vi "Puzzle 7-1.vi"() -> ()   [LabVIEW 2022 SP3]
uses:
  <vilib>/Analysis/NI_AALBase.lvlib
panel:
  in  "delimited string":string="Time:        53     71     78     80\nDistance:   275   1181   1215   1524"
  out "Numeric":i64
  out "Array":T1(array[ring])
  out "logical OR":bool
  out "Hands sorted":T2(array[cluster])
  out "Hands identified":T2(array[cluster])
  out "Map":map{string, u8}(c390)
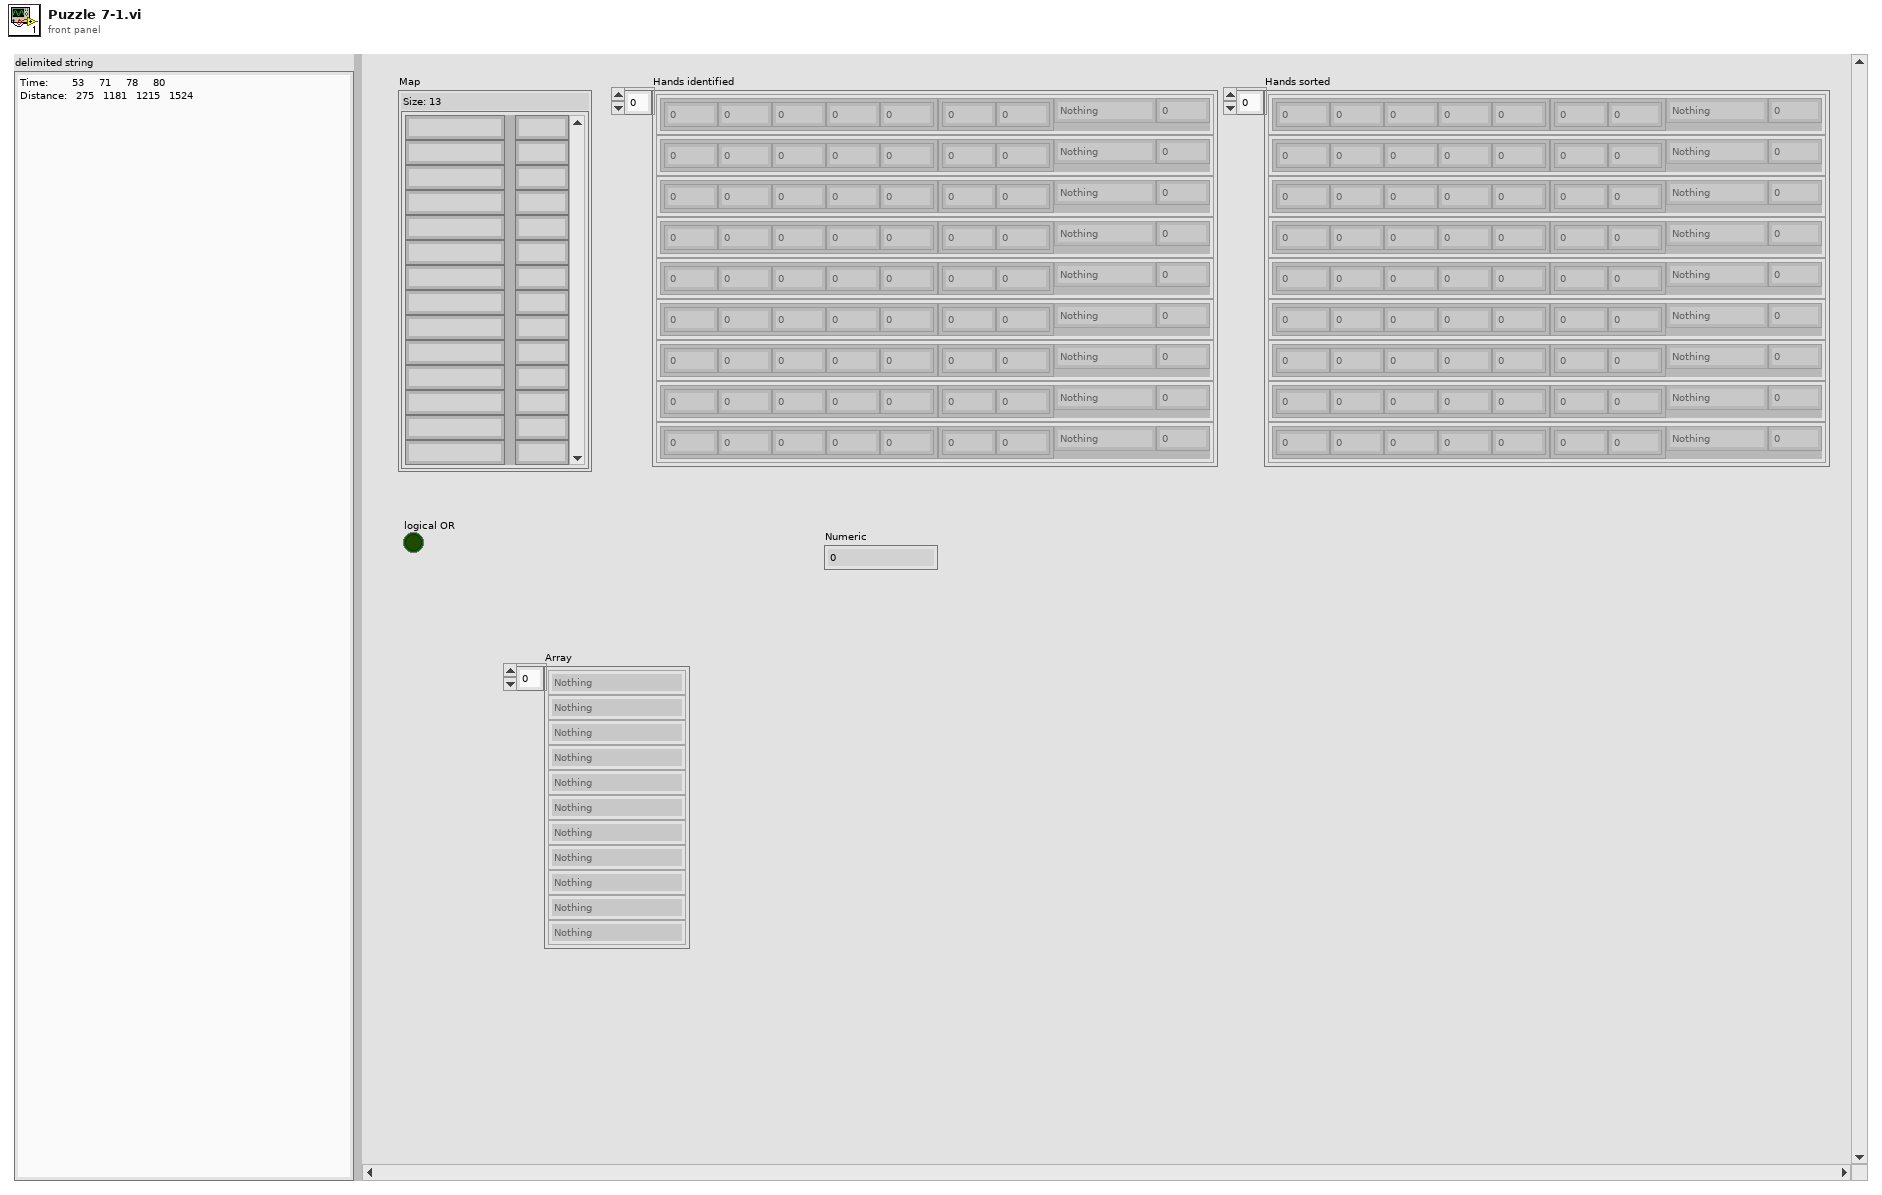
[diagram p1: front panel]
types:
  T1 = enum16{"Nothing", "One Pair", "Two Pair", "Three of a Kind", "Full House", "Four of a Kind", "Five of a Kind"}[]
  T2 = cluster{u8[], cluster{"size":i32, i32}, "value":enum16{"Nothing", "One Pair", "Two Pair", "Three of a Kind", "Full House", "Four of a Kind", "Five of a Kind"}, i32}[]
  T3 = map{enum16{"Nothing", "One Pair", "Two Pair", "Three of a Kind", "Full House", "Four of a Kind", "Five of a Kind"}, set{cluster{u8[], cluster{"size":i32, i32}, "value":enum16{"Nothing", "One Pair", "Two Pair", "Three of a Kind", "Full House", "Four of a Kind", "Five of a Kind"}, i32}}}
  T4 = enum16{"Nothing", "One Pair", "Two Pair", "Three of a Kind", "Full House", "Four of a Kind", "Five of a Kind"}
  T5 = map{cluster{"size of set":i32, "histogram max":i32}, enum16{"Nothing", "One Pair", "Two Pair", "Three of a Kind", "Full House", "Four of a Kind", "Five of a Kind"}}
  T6 = cluster{u8[], cluster{"size":i32, i32}, "value":enum16{"Nothing", "One Pair", "Two Pair", "Three of a Kind", "Full House", "Four of a Kind", "Five of a Kind"}, i32}
  T7 = set{cluster{u8[], cluster{"size":i32, i32}, "value":enum16{"Nothing", "One Pair", "Two Pair", "Three of a Kind", "Full House", "Four of a Kind", "Five of a Kind"}, i32}}
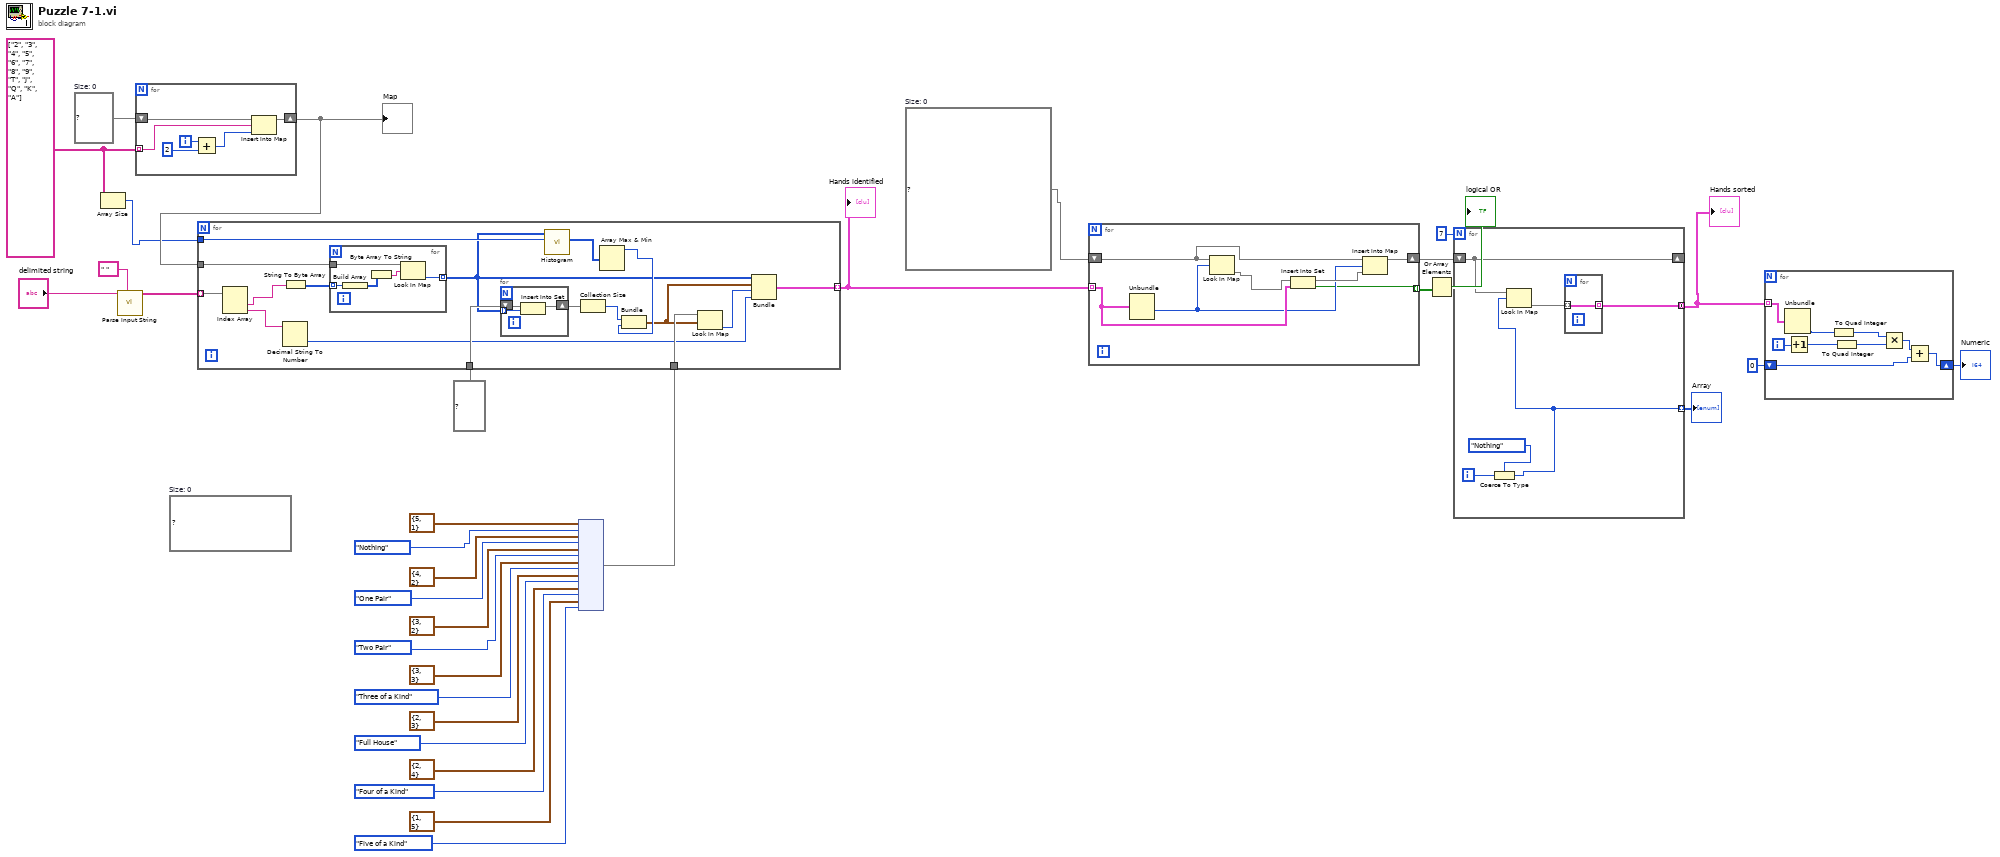
[diagram p0: block diagram]
diagram:
  w10 = T3 {}  # Size: 0
  (unwired) T5 {}  # Size: 0
  w30 = map{string, u8} {}  # Size: 0
  w27 = string[] ["2", "3", "4", "5", "6", "7", "8", "9", "T", "J", "Q", "K", "A"]
  n1 = Array Size(array=w27) -> (size(s)=w26:i32)
  n2 = call "Parse Input String.vi"("delimiter (Tab)"=" ", "delimited string"="delimited string") -> ("parsed string"=w31:string[][])  [unwired: 9 in]
  n3 = for {
    tunnel: w27 -> [w37] mode=indexing
    shift-right: [w38] -> w29
    shift-left: w30 -> [w39]
    i -> [w36]
    n4 = Add(x=w36, y=2) -> (x+y=w34:i32)
    n5 = Insert Into Map(map in=w39, key=w37, value=w34) -> (map out=w38:map{string, u8})  [unwired: 2 out]
  }
  "Map" <- w29
  n6 = node(cluster{"size of set":i32, "histogram max":i32} {"size of set"=5, "histogram max"=1}, T4."Nothing", cluster{"size of set":i32, "histogram max":i32} {"size of set"=4, "histogram max"=2}, T4."One Pair", cluster{"size of set":i32, "histogram max":i32} {"size of set"=3, "histogram max"=2}, T4."Two Pair", cluster{"size of set":i32, "histogram max":i32} {"size of set"=3, "histogram max"=3}, T4."Three of a Kind", cluster{"size of set":i32, "histogram max":i32} {"size of set"=2, "histogram max"=3}, T4."Full House", cluster{"size of set":i32, "histogram max":i32} {"size of set"=2, "histogram max"=4}, T4."Four of a Kind", cluster{"size of set":i32, "histogram max":i32} {"size of set"=1, "histogram max"=5}, T4."Five of a Kind") -> (w9:T5)
  n7 = for {
    tunnel: w31 -> [w56] mode=indexing
    tunnel: w29 -> [w54]
    tunnel: set{u8} {} ("set in") -> [w51]
    tunnel: w26 -> [w49]
    tunnel: w9 -> [w45]
    tunnel: [w40] -> w11 mode=indexing
    n8 = Index Array(array=w56) -> (element #1=w53:string, element #2=w55:string)  [unwired: 2 in]
    n9 = Decimal String To Number(string=w55) -> (number=w41:i32)  [unwired: 2 in, 1 out]
    n10 = String To Byte Array(string=w53) -> (unsigned byte array=w52:u8[])
    n11 = for {
      tunnel: w54 -> [w64]
      tunnel: [w63] -> w44 mode=indexing
      tunnel: w52 -> [w62] mode=indexing
      n12 = Build Array(w62) -> (w61:u8[])
      n13 = Byte Array To String(unsigned byte array=w61) -> (string=w60:string)
      n14 = Look In Map(map=w64, key=w60) -> (value=w63:u8)  [unwired: 1 in, 1 out]
    }
    n15 = for {
      tunnel: w44 -> [w59] mode=indexing
      shift-right: [w57] -> w50
      shift-left: w51 -> [w58]
      n16 = Insert Into Set(10:w59, 11:w58) -> (3:w57:set{u8})  [unwired: 1 out]
    }
    n17 = call <vilib>:"Histogram.vi"("intervals"=w49, "X"=w44) -> ("Histogram: h(x)"=w47:i32[])  [unwired: 6 in, 3 out]
    n18 = Collection Size(1:w50) -> (0:w48:i32)
    n19 = Array Max & Min(array=w47) -> (max value=w46:i32)  [unwired: 3 out]
    n20 = Bundle("size"=w48, w46) -> (w43:cluster{"size":i32, i32})  [unwired: 1 in]
    n21 = Look In Map(map=w45, key=w43) -> (value=w42:T4)  [unwired: 1 in, 1 out]
    n22 = Bundle(w44, w43, "value"=w42, w41) -> (w40:T6)  [unwired: 1 in]
  }
  "Hands identified" <- w11
  n23 = for {
    tunnel: w11 -> [w70] mode=indexing
    shift-right: [w66] -> w8
    shift-left: w10 -> [w69]
    tunnel: [w65] -> w7 mode=indexing
    n24 = Unbundle(w70) -> ("value"=w67:T4)  [unwired: 3 out]
    n25 = Look In Map(map=w69, key=w67) -> (value=w71:T7)  [unwired: 1 in, 1 out]
    n26 = Insert Into Set(10:w70, 11:w71) -> (2:w65:bool, 3:w68:T7)
    n27 = Insert Into Map(map in=w69, key=w67, value=w68) -> (map out=w66:T3)  [unwired: 2 out]
  }
  n28 = Or Array Elements(Boolean array=w7) -> (logical OR=→"logical OR":bool)
  n29 = for {
    N: 7 -> [_]
    shift-right: [w76] -> _
    shift-left: w8 -> [w76]
    tunnel: [w75] -> w3 mode=concatenating
    tunnel: [w72] -> w5 mode=indexing
    i -> [w74]
    n30 = Coerce To Type(0:w74, 1:T4."Nothing" ("value")) -> (2:w72:T4)
    n31 = Look In Map(map=w76, key=w72) -> (value=w77:T7)  [unwired: 1 in, 1 out]
    n32 = for {
      tunnel: w77 -> [w78] mode=indexing
      tunnel: [w78] -> w75 mode=indexing
    }
  }
  "Hands sorted" <- w3
  "Array" <- w5
  n33 = for {
    tunnel: w3 -> [w86] mode=indexing
    shift-right: [w82] -> w1
    shift-left: i64 0 -> [w81]
    i -> [w87]
    n34 = Unbundle(w86) -> (w85:i32)  [unwired: 3 out]
    n35 = Increment(x=w87) -> (x+1=w84:i32)
    n36 = To Quad Integer(1:w85) -> (0:w80:i64)
    n37 = To Quad Integer(1:w84) -> (0:w79:i64)
    n38 = Multiply(x=w80, y=w79) -> (x*y=w83:i64)
    n39 = Add(x=w83, y=w81) -> (x+y=w82:i64)
  }
  "Numeric" <- w1
